vi "Read_DI_2_CVT.vi"() -> ()   [LabVIEW 2016]
uses:
  <vilib>/NI/Current Value Table/DataTypes/Boolean_Read.vi
  <vilib>/NI/Current Value Table/Type to Enum.vi
  <vilib>/NI/Current Value Table/DataTypes/Boolean_Type To Enum.vi
  <vilib>/Utility/file.llb/Read Delimited Spreadsheet (string).vi
  <vilib>/NI/Current Value Table/FGVs/CVT Globals.vi
  <vilib>/NI/Current Value Table/FGVs/Tag Memory.vi
  <vilib>/NI/Current Value Table/Memory Block.vi
  <vilib>/NI/Current Value Table/DataTypes/Boolean_Memory Block.vi
  <vilib>/NI/Current Value Table/Current Value Table.lvlib
panel:
  in  "Cancel Button":bool
  out "subarray 3":cluster{bool}[](array[cluster])
  out "subarray":cluster{bool}[](array[cluster])
  # "DOORS FB AND SENSOR\n                                  STATUS"
  # "Spare DI-2"
  # "OT Entrance-Hand Santizier Proxy"
  # "Ist O.T-AHU Run FB"
  # "Spare DI-1"
  # "2nd O.T-Scrubber Proxy"
  # "OT Entrance-Door Inside Open PB"
  # "2nd O.T-Door Inside Open PB"
  # "OT Entrance-Door Open Proxy FB"
  # "2nd O.T-Door Open Proxy FB"
  # "Ist O.T -Scrubber Proxy"
  # "Ist O.T-E-Stop PB"
  # "Ist O.T-Door Inside Open PB"
  # "2nd O.T-E-Stop PB"
  # "Ist O.T-Door  Open Proxy FB"
  # "DOORS FB AND SENSOR\n                                  STATUS"
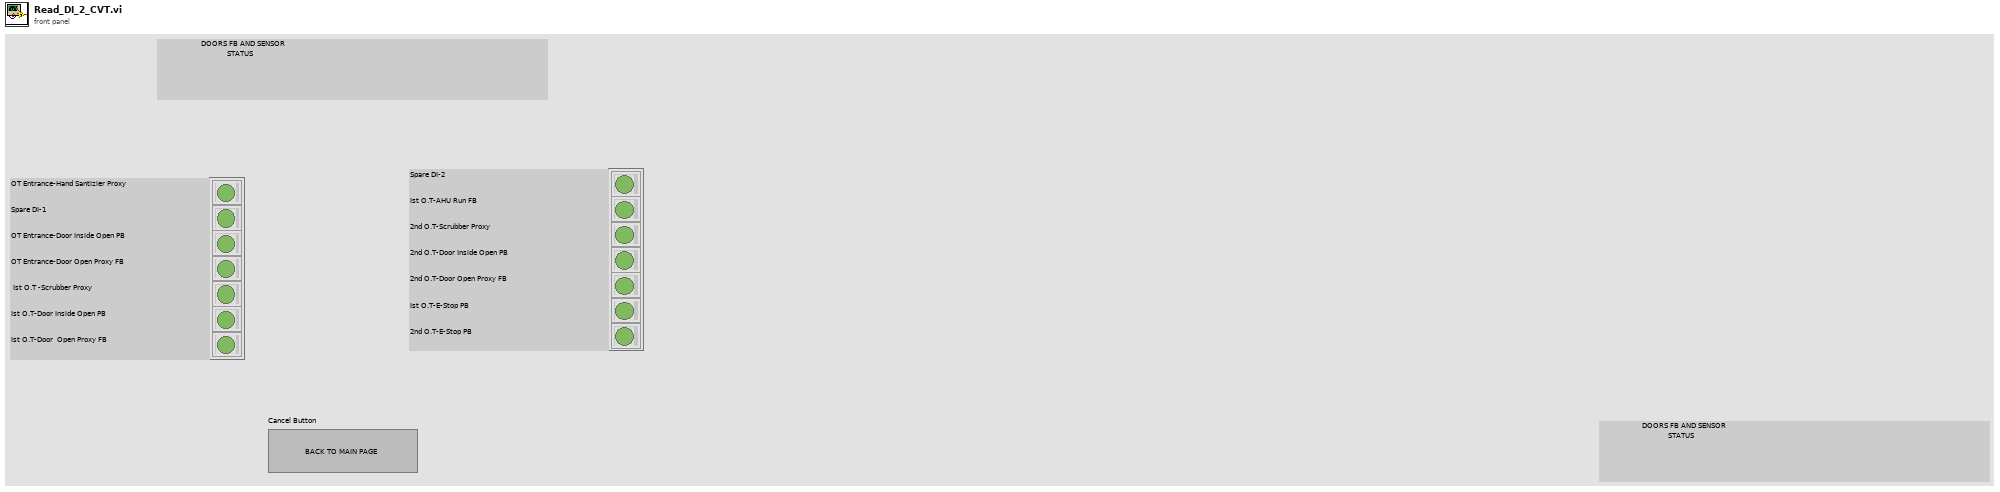
[diagram p1: front panel]
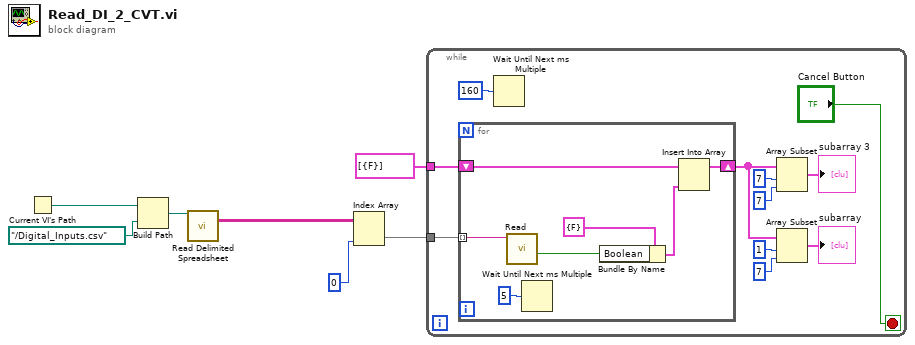
[diagram p0: block diagram]
diagram:
  n1 = Current VI's Path() -> (path=w3:path)
  n2 = Build Path(base path=w3, name or relative path=path "../Digital_Inputs.csv") -> (appended path=w1:path)
  n3 = call-poly <vilib>:"Read Delimited Spreadsheet.vi"("file path (dialog if empty)"=w1) -> ("all rows"=w6:string[][])  [unwired: 9 in, 5 out]
  n4 = Index Array "Index Array"(array=w6, index (col)=0 ("disabled index (col)")) -> (element=w4:string[])  [unwired: 1 in]
  n5 = while {
    tunnel: cluster{"Boolean":bool}[] [{"Boolean"=FALSE}] ("output array") -> [w18]
    tunnel: w4 -> [w17]
    stop <- "Cancel Button" stop-if-true
    n6 = for {
      shift-right: [w22] -> w14
      shift-left: w18 -> [w23]
      tunnel: w17 -> [w21] mode=indexing
      n7 = call-poly <vilib>:"Read.vi"("Tag Name"=w21) -> ("Value"=w20:bool)  [unwired: 9 in, 1 out]
      n8 = Wait Until Next ms Multiple(millisecond multiple=u32 5 ("millisecond timer value")) -> ()  [unwired: 1 out]
      n9 = Bundle By Name(cluster=cluster{"Boolean":bool} {"Boolean"=FALSE} ("Cluster"), "Boolean"=w20) -> (w24:cluster{"Boolean":bool})
      n10 = Insert Into Array(array=w23, new element=w24) -> (w22:cluster{"Boolean":bool}[])  [unwired: 1 in]
    }
    n11 = Wait Until Next ms Multiple(millisecond multiple=u32 160) -> ()  [unwired: 1 out]
    n12 = Array Subset(array=w14, index=7, length=7) -> (→"subarray 3":cluster{"Boolean":bool}[])
    n13 = Array Subset(array=w14, index=1, length=7) -> (→"subarray":cluster{"Boolean":bool}[])
  }
